vi "Problem2.5.vi"() -> ()   [LabVIEW 2019]
panel:
  out "Time Between Loop Iterations":dbl
  in  "ms to Wait":dbl=50.0
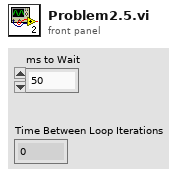
[diagram p1: front panel]
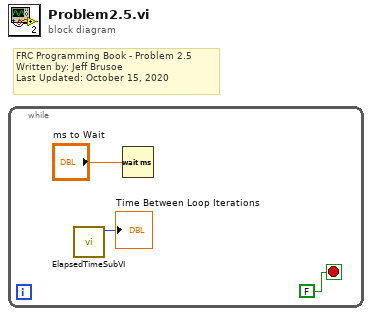
[diagram p0: block diagram]
diagram:
  # "FRC Programming Book - Problem 2.5\nWritten by: Jeff Brusoe\nLast Updated: October 15, 2020"
  n1 = while {
    stop <- FALSE stop-if-true
    n2 = call "ElapsedTimeSubVI.vi"() -> ("Numeric"=→"Time Between Loop Iterations":u32)  [unwired: 11 in]
    n3 = Wait (ms)(milliseconds to wait="ms to Wait") -> ()  [unwired: 1 out]
  }
